vi "Auto-Write to Folder and file for LaserPD_YCC.vi"(4 "Who's Data":enum16{"YCC", "PYW", "LCH", "YYH"}(ring), 5 "T=2D\nF=1D":bool=TRUE, 6 "2D data to be saved":dbl[][](array[numeric]) format="%0.2f", 7 "1D data to be saved":dbl[](array[numeric]) format="%0.2f", 8 "File name add to the end \n(height)":string="h300", 9 "Save?":bool) -> (2 "Save to File Name":string, 3 "Save to Path":path)   [LabVIEW 2014]
uses:
  Main-Stage-PI/(Global) Current handle and LaserPower_YCC.vi
  <vilib>/Utility/file.llb/Write To Spreadsheet File (DBL).vi
panel:
  out "Folder name":string
  out "folder exists?":bool
  out "date/time string":string
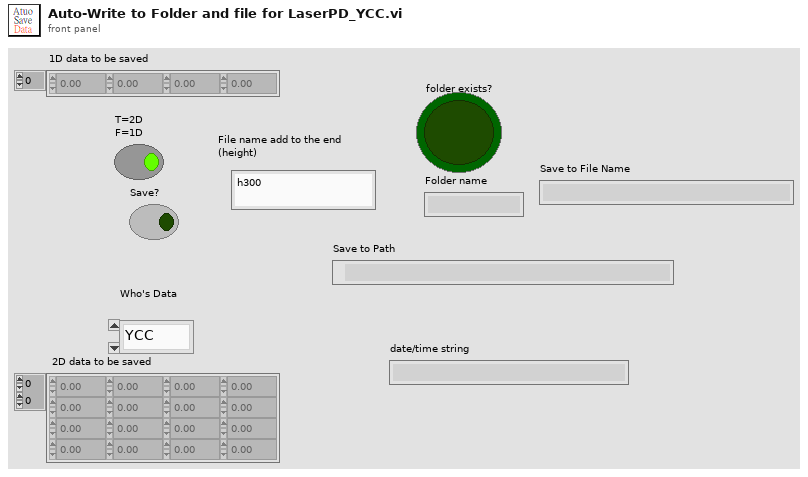
[diagram p1: front panel]
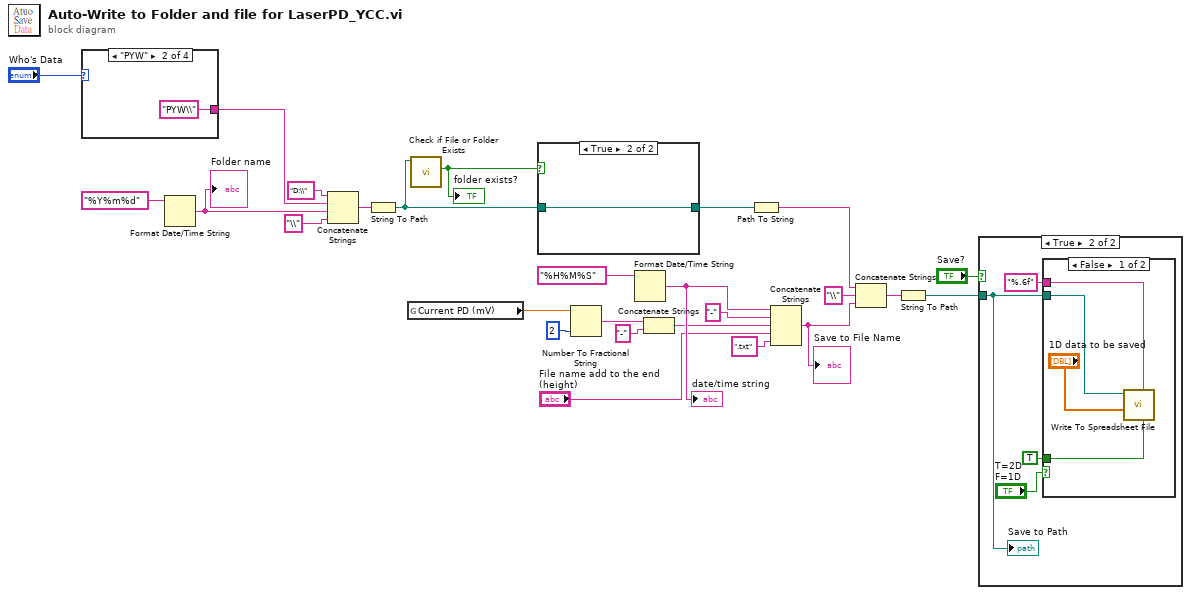
[diagram p0: block diagram]
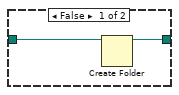
[diagram p2: hidden frame]
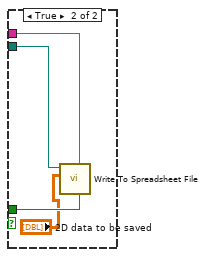
[diagram p4: hidden frame]
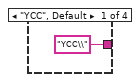
[diagram p5: hidden frame]
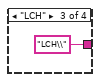
[diagram p6: hidden frame]
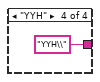
[diagram p7: hidden frame]
diagram:
  n1 = case shown="\"PYW\"" "Who's Data" {
    tunnel: ["YCC\\" ("string") "PYW\\" ("string") "LCH\\" ("string") "YYH\\" ("string")] -> w24
    frame "YCC", Default {
    }
    frame "PYW" {
    }
    frame "LCH" {
    }
    frame "YYH" {
    }
  }
  n2 = Format Date/Time String(time format string (%c)="%Y%m%d") -> (date/time string=w11:string)  [unwired: 2 in]
  "Folder name" <- w11
  n3 = Concatenate Strings("D:\\" ("string"), w24, w11, "\\" ("string")) -> (w23:string)
  n4 = String To Path(string=w23) -> (path=w14:path)
  n5 = global read "(Global) Current handle and LaserPower_YCC.vi" "Current PD (mV)"() -> (w6:dbl)
  n6 = call <vilib>:"Check if File or Folder Exists.vi"("path"=w14) -> ("file or folder exists?"=w13:bool)  [unwired: 8 in, 2 out]
  "folder exists?" <- w13
  n7 = case shown="True" w13 {
    tunnel: w14 -> [w32 w33]
    tunnel: [w31 w33] -> w19
    frame False {
      n8 = Create Folder(path (use dialog)=w32) -> (created path=w31:path)  [unwired: 2 in, 2 out]
    }
    frame True {
    }
  }
  n9 = Number To Fractional String(number=w6, precision (6)=i16 2) -> (F-format string=w4:string)  [unwired: 2 in]
  n10 = Format Date/Time String(time format string (%c)="%H%M%S") -> (date/time string=w9:string)  [unwired: 2 in]
  "date/time string" <- w9
  n11 = Concatenate Strings(w4, "-" ("string")) -> (w2:string)
  n12 = Path To String(path=w19) -> (string=w16:string)
  n13 = Concatenate Strings(w9, "-" ("string"), w2, "File name add to the end \n(height)", ".txt" ("string")) -> (w10:string)
  "Save to File Name" <- w10
  n14 = Concatenate Strings(w16, "\\" ("string"), w10) -> (w18:string)
  n15 = String To Path(string=w18) -> (path=w17:path)
  n16 = case shown="True" "Save?" {
    tunnel: w17 -> [_ w36]
    frame False {
    }
    frame True {
      n17 = case shown="False" "T=2D\nF=1D" {
        tunnel: TRUE ("transpose? (no:F)") -> [w38 w45]
        tunnel: w36 -> [w40 w44]
        tunnel: "%.6f" ("format (%.3f)") -> [w41 w43]
        frame False {
          n18 = call-poly <vilib>:"Write To Spreadsheet File.vi"("transpose? (no:F)"=w38, "format (%.3f)"=w41, "1D data"="1D data to be saved", "file path (dialog if empty)"=w40) -> ()  [unwired: 4 in, 1 out]
        }
        frame True {
          n19 = call-poly <vilib>:"Write To Spreadsheet File.vi"("transpose? (no:F)"=w45, "format (%.3f)"=w43, "2D data"="2D data to be saved", "file path (dialog if empty)"=w44) -> ()  [unwired: 4 in, 1 out]
        }
      }
      "Save to Path" <- w36
    }
  }
